vi "Save Setting.vi"(8 "error in (no error)":errorcluster, 11 "FW102C in":i32) -> (0 "error out":errorcluster, 3 "FW102C out":i32)   [LabVIEW 2017, in "Colour Wheel.lvlib" / "Thorlabs_FW102C.lvlib"]
doc: "This will save all the settings as default on power up"
uses:
  Thorlabs_FW102C.lvlib
  Library/FilterWheel102_win32.dll
  Library/FilterWheel102_win64.dll
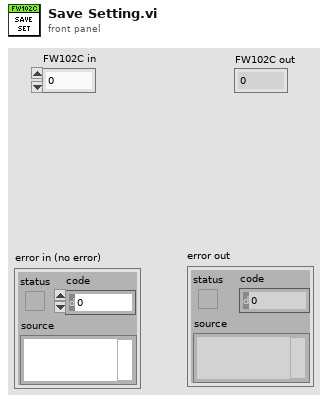
[diagram p1: front panel]
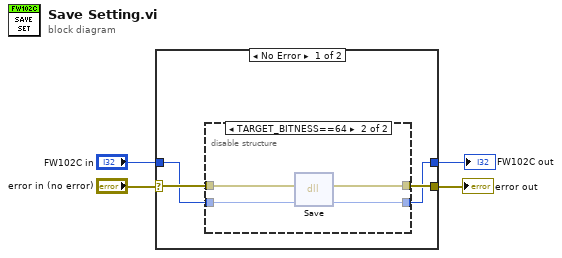
[diagram p0: block diagram]
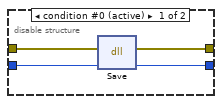
[diagram p2: hidden frame]
diagram:
  n1 = case shown="No Error" "error in (no error)" {
    selector: "error in (no error)" -> [w8 w17]
    tunnel: [w7 w17] -> w4
    tunnel: "FW102C in" -> [w6 w18]
    tunnel: [w5 w18] -> w1
    frame No Error {
      n2 = disable-structure shown="TARGET_BITNESS==64" {
        disable-tunnel: w8 -> [w12 w16]
        disable-tunnel: [w11 w15] -> w7
        disable-tunnel: w6 -> [w10 w14]
        disable-tunnel: [w9 w13] -> w5
        frame condition #0 (active) {
          n3 = dll-call lib="C:/Project Work/icl-optical-software-rewrite/Optical Software Code Simplified/Modules/Colour Wheel/Thorlabs_FW102C/Library/FilterWheel102_win32.dll" fn="Save"(error in=w12, "hdl"=w10) -> (error out=w11:errorcluster, "hdl"=w9:i32)  [unwired: 3 in, 1 out]
        }
        frame condition #1 {
          n4 = dll-call lib="C:/Project Work/icl-optical-software-rewrite/Optical Software Code Simplified/Modules/Colour Wheel/Thorlabs_FW102C/Library/FilterWheel102_win64.dll" fn="Save"(error in=w16, "hdl"=w14) -> (error out=w15:errorcluster, "hdl"=w13:i32)  [unwired: 3 in, 1 out]
        }
      }
    }
    frame Error {
    }
  }
  "error out" <- w4
  "FW102C out" <- w1
